vi "FITS Filter Name.vi"(8 "error in (no error)":errorcluster, 11 "Hdr Name":string) -> (0 "error out":errorcluster, 3 "Filtered Name":string)   [LabVIEW 2024]
uses:
  <vilib>/Utility/error.llb/Trim Whitespace One-Sided.vi
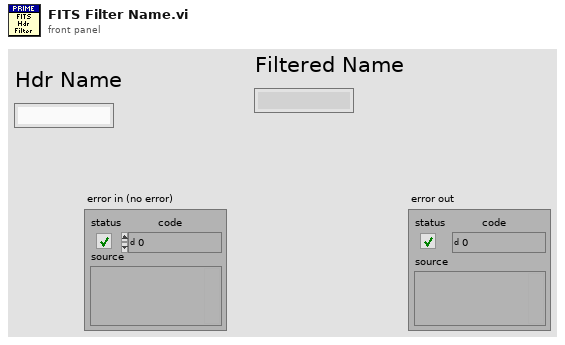
[diagram p1: front panel]
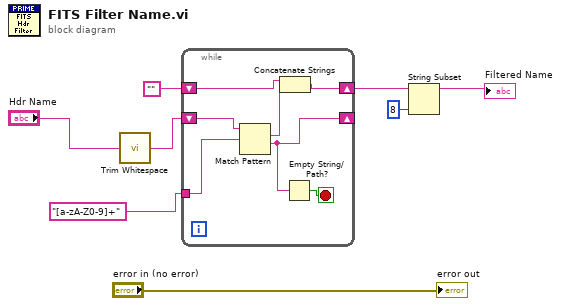
[diagram p0: block diagram]
diagram:
  n1 = call <vilib>:"Trim Whitespace.vi"("string"="Hdr Name") -> ("trimmed string"=w1:string)  [unwired: 1 in]
  n2 = while {
    shift-right: [w11] -> w7
    shift-left: "" -> [w10]
    tunnel: "[a-zA-Z0-9]+" ("regular expression") -> [w12]
    shift-right: [w9] -> _
    shift-left: w1 -> [w15]
    stop <- w13 stop-if-true
    n3 = Match Pattern(string=w15, regular expression=w12) -> (match substring=w14:string, after substring=w9:string)  [unwired: 1 in, 2 out]
    n4 = Concatenate Strings(w10, w14) -> (w11:string)
    n5 = Empty String/Path?(string/path=w9) -> (empty?=w13:bool)
  }
  n6 = String Subset(string=w7, length (rest)=8 ("length (rest)")) -> (substring=→"Filtered Name":string)  [unwired: 1 in]
  "error out" <- "error in (no error)"
